vi "删除小跳跃点.vi"(2 "数组－数值 2":dbl[](array[numeric]), 3 "数组－数值":dbl[](array[numeric])) -> (0 "第二列":dbl[](array[numeric]), 1 "第一列":dbl[](array[numeric]))   [LabVIEW 2016]
panel:
  in  "数组 4":dbl[](array[numeric])
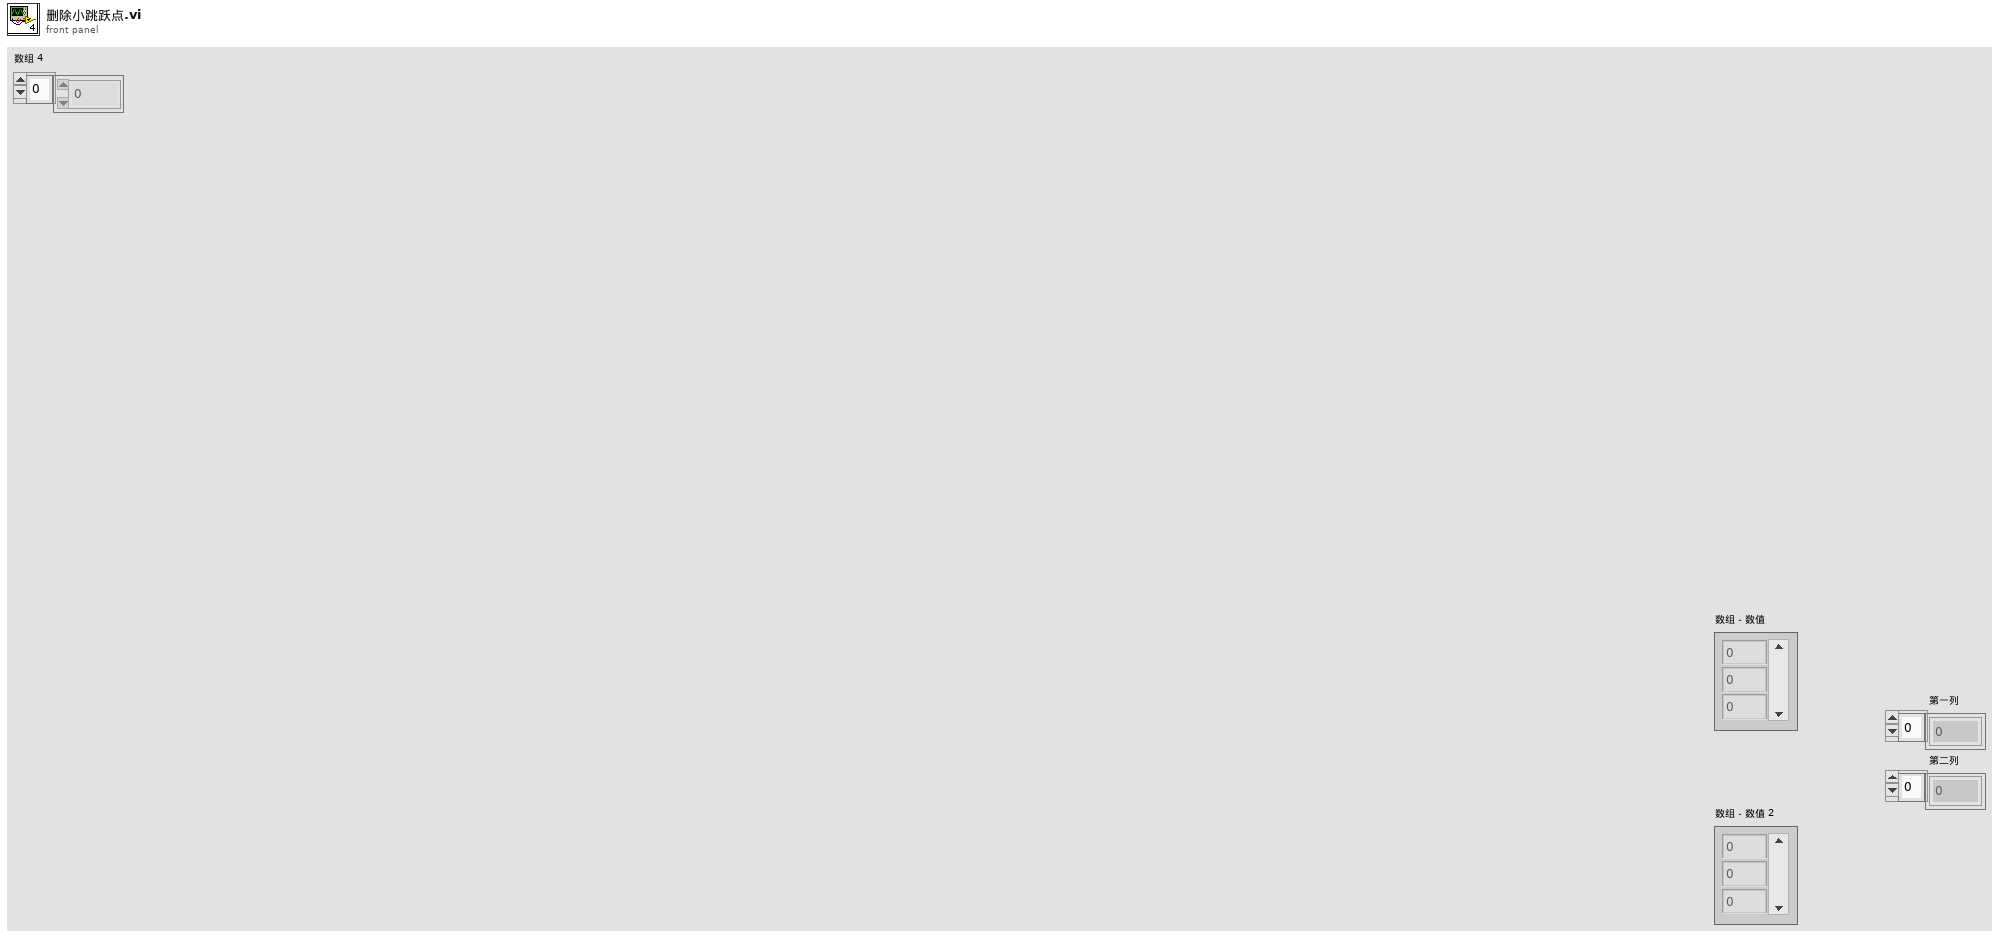
[diagram p1: front panel]
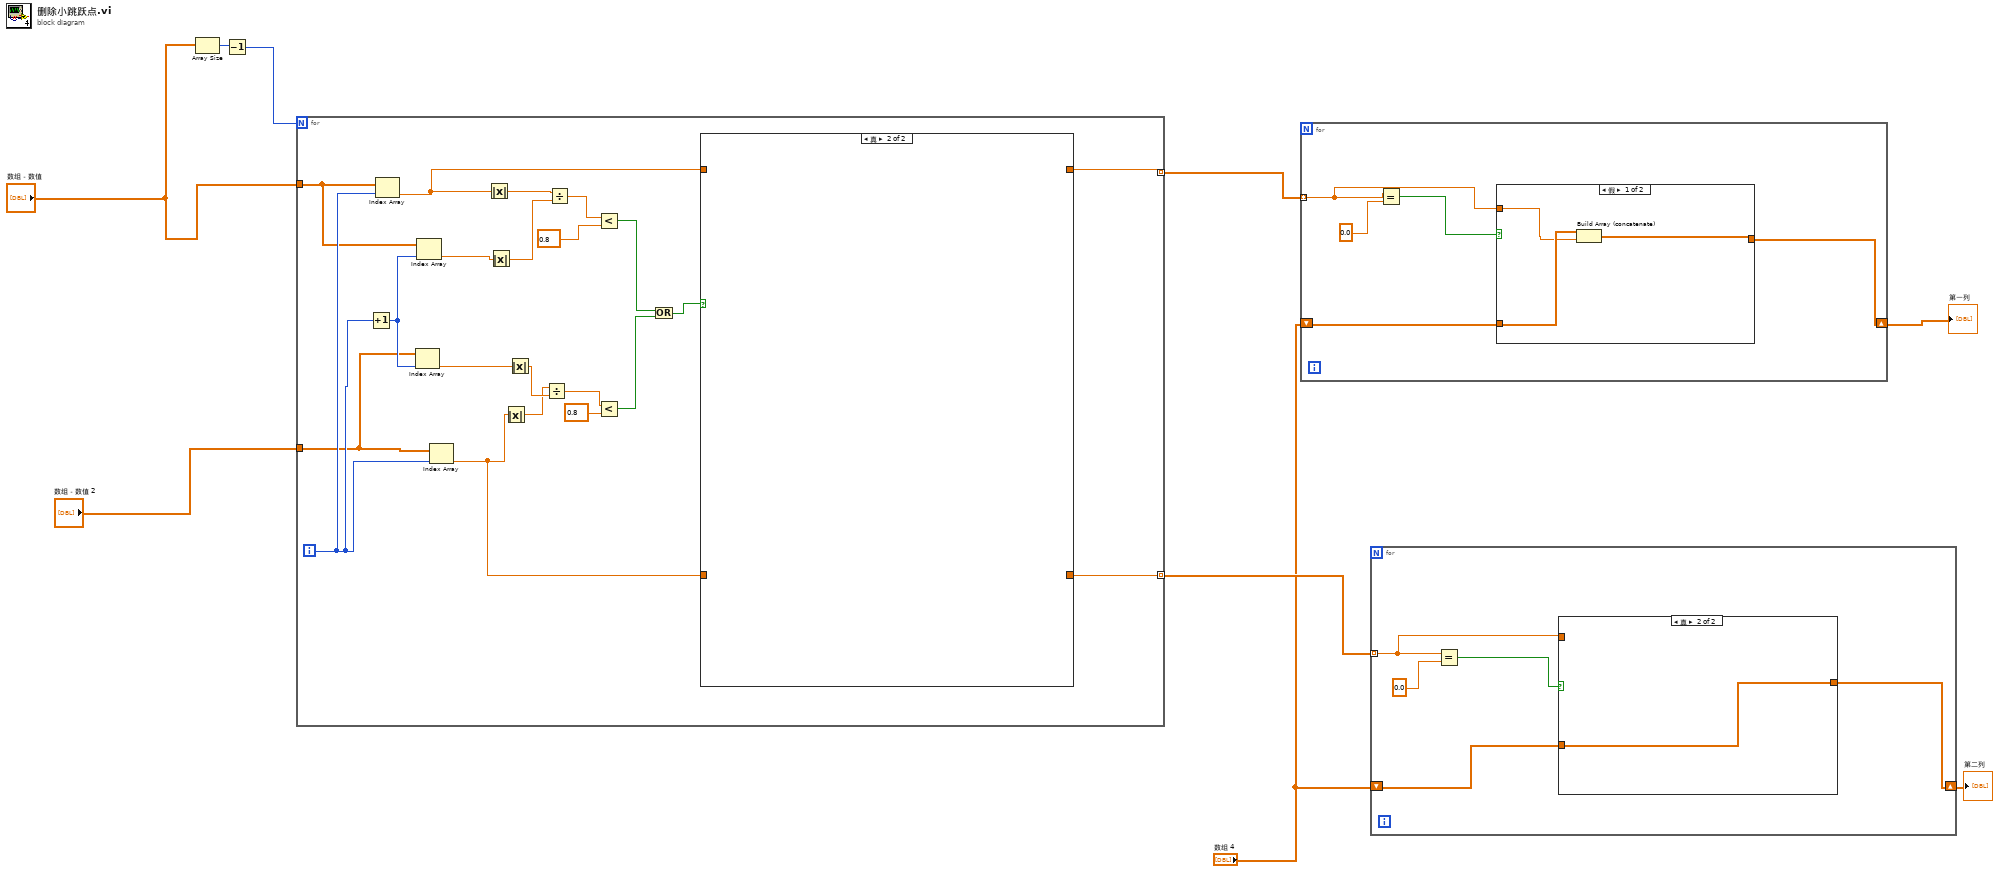
[diagram p0: block diagram]
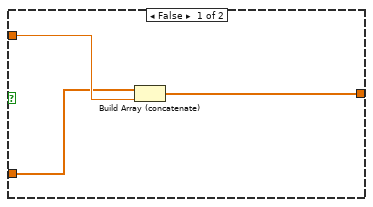
[diagram p2: hidden frame]
diagram:
  n1 = Array Size(array="数组－数值") -> (size(s)=w9:i32)
  n2 = Decrement(x=w9) -> (x-1=w8:i32)
  n3 = for {
    N: w8 -> [_]
    tunnel: "数组－数值" -> [w28]
    tunnel: "数组－数值 2" -> [w27]
    tunnel: [w19] -> w7 mode=indexing
    tunnel: [w18] -> w6 mode=indexing
    i -> [w30]
    n4 = Increment(x=w30) -> (x+1=w29:i32)
    n5 = Index Array(array=w28, index=w30) -> (element=w17:dbl)
    n6 = Index Array(array=w27, index=w29) -> (element=w15:dbl)
    n7 = Index Array(array=w28, index=w29) -> (element=w16:dbl)
    n8 = Index Array(array=w27, index=w30) -> (element=w14:dbl)
    n9 = Absolute Value(x=w17) -> (abs(x)=w13:dbl)
    n10 = Absolute Value(x=w16) -> (abs(x)=w12:dbl)
    n11 = Absolute Value(x=w14) -> (abs(x)=w10:dbl)
    n12 = Absolute Value(x=w15) -> (abs(x)=w11:dbl)
    n13 = Divide(x=w10, y=w11) -> (x/y=w24:dbl)
    n14 = Divide(x=w13, y=w12) -> (x/y=w26:dbl)
    n15 = Less?(x=w26, y=0.8) -> (x < y?=w22:bool)
    n16 = Less?(x=w24, y=0.8) -> (x < y?=w21:bool)
    n17 = Or(x=w22, y=w21) -> (x .or. y?=w20:bool)
    n18 = case shown="真" w20 {
      tunnel: w17 -> [w32 _]
      tunnel: w14 -> [w31 _]
      tunnel: [w32 _] -> w19
      tunnel: [w31 _] -> w18
      frame False {
      }
      frame True {
      }
    }
  }
  n19 = for {
    tunnel: w7 -> [w35] mode=indexing
    shift-right: [w33] -> w2
    shift-left: "数组 4" -> [w34]
    n20 = Equal?(x=w35, y=0.0) -> (x = y?=w36:bool)
    n21 = case shown="假" w36 {
      tunnel: w35 -> [w38 _]
      tunnel: w34 -> [w39 w41]
      tunnel: [w40 w41] -> w33
      frame False {
        n22 = Build Array (concatenate)(w39, w38) -> (w40:dbl[])
      }
      frame True {
      }
    }
  }
  "第一列" <- w2
  n23 = for {
    tunnel: w6 -> [w44] mode=indexing
    shift-right: [w42] -> w1
    shift-left: "数组 4" -> [w43]
    n24 = Equal?(x=w44, y=0.0) -> (x = y?=w45:bool)
    n25 = case shown="真" w45 {
      tunnel: w44 -> [w49 _]
      tunnel: w43 -> [w48 w50]
      tunnel: [w47 w50] -> w42
      frame False {
        n26 = Build Array (concatenate)(w48, w49) -> (w47:dbl[])
      }
      frame True {
      }
    }
  }
  "第二列" <- w1
